vi "DAQmx(AI).ReftoDVR.vi"(10 "Ref":u32 format="%08x") -> (2 "Ref":T1)   [LabVIEW 2013, in "DAQmx(AI).lvclass"]
doc: "JKI State Machine Objects (SMO) 1.0.0.5\nJKI - JKI\nCopyright (c) 2016, JKI"
uses:
  DAQmx(AI).lvclass
  Typedefs/PrivateData--Ref.ctl
  Typedefs/PrivateData--Cluster.ctl
  Typedefs/Configuration--Cluster.ctl
  Typedefs/Units -- Enum.ctl
  Typedefs/PublicEvents--Cluster.ctl
  Typedefs/DataChanged--EventData--Cluster.ctl
  Typedefs/ScalingEvent--Cluster.ctl
  Typedefs/Scaling(MapRange)--Cluster.ctl
  Typedefs/Scaling--Cluster.ctl
  Typedefs/ScalingType--Enum.ctl
  Typedefs/Scaling(Linear)--Cluster.ctl
  Typedefs/Scaling(Polynomial)--Cluster.ctl
  Typedefs/Scaling(Table)--Cluster.ctl
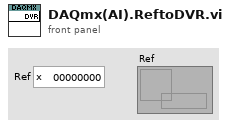
[diagram p1: front panel]
types:
  T1 = typedef "DAQmx(AI).lvclass/PrivateData--Ref.ctl" = refnum<data-value>
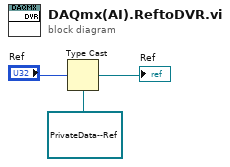
[diagram p0: block diagram]
diagram:
  n1 = Type Cast(type=T1 refnum ("Ref"), x="Ref") -> (*(type *) &x=→"Ref":T1)
